vi "HoodPID.vi"(4 "Deadband":dbl, 5 "TAReset":bool, 6 "TAGains":T1={"proportional gain (Kc)"=1.0, "integral time (Ti, min)"=0.01, "derivative time (Td, min)"=0.0} {"derivative time (Td, min)" format="%.3f"; "integral time (Ti, min)" format="%.3f"; "proportional gain (Kc)" format="%.3f"}, 7 "TARange":cluster{"output high":dbl, "output low":dbl}={"output high"=0.6, "output low"=-0.6} {"output low" format="%.2f"; "output high" format="%.2f"}, 8 "TADisable Range":dbl, 9 "TAIntegral Range":dbl=10000.0, 10 "TAProcess variable":dbl, 11 "TASetpoint":dbl) -> (2 "TAoutput":dbl format="%.2f")   [LabVIEW 2020]
uses:
  <vilib>/addons/control/pid/pid.llb/PID (DBL).vi
  <vilib>/addons/control/pid/NI_PID_pid.lvlib
panel:
  out "TAChart":cluster{"Setpoint":dbl, "Process variable":dbl}(graph)
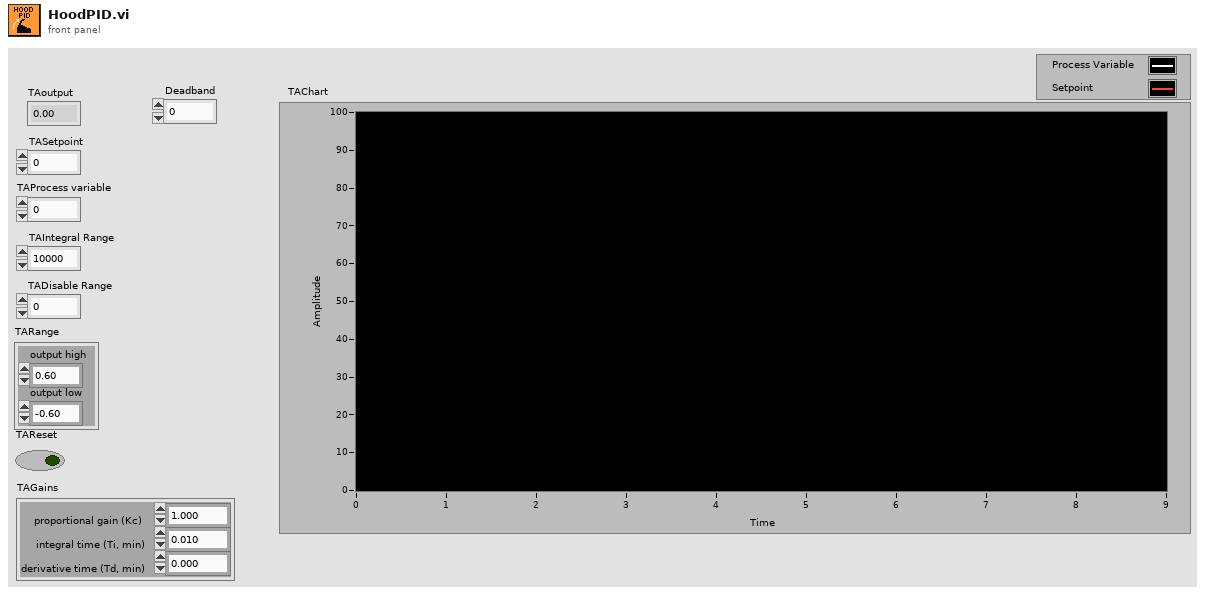
[diagram p1: front panel]
types:
  T1 = cluster{"proportional gain (Kc)":dbl, "integral time (Ti, min)":dbl, "derivative time (Td, min)":dbl}
  T2 = cluster{"TASetpoint":dbl, "TAProcess variable":dbl}
  T3 = cluster{"proportional gain (Kc)":dbl, "f":dbl, "derivative time (Td, min)":dbl}
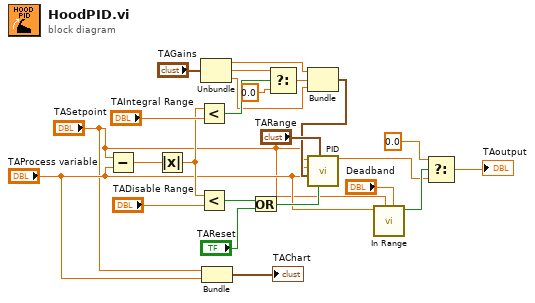
[diagram p0: block diagram]
diagram:
  n1 = Subtract(x="TASetpoint", y="TAProcess variable") -> (x-y=w23:dbl)
  n2 = Absolute Value(x=w23) -> (abs(x)=w13:dbl)
  n3 = Less?(x=w13, y="TAIntegral Range") -> (x < y?=w21:bool)
  n4 = Less?(x=w13, y="TADisable Range") -> (x < y?=w11:bool)
  n5 = Unbundle("TAGains") -> ("proportional gain (Kc)"=w16:dbl, "integral time (Ti, min)"=w19:dbl, "derivative time (Td, min)"=w15:dbl)
  n6 = Bundle("TASetpoint"="TASetpoint", "TAProcess variable"="TAProcess variable") -> (→"TAChart":T2)  [unwired: 1 in]
  n7 = Or(x=w11, y="TAReset") -> (x .or. y?=w10:bool)
  n8 = Select(t=w19, s=w21, f=0.0) -> (s? t:f=w17:dbl)
  n9 = Bundle("proportional gain (Kc)"=w16, "f"=w17, "derivative time (Td, min)"=w15) -> (w9:T3)  [unwired: 1 in]
  n10 = call-poly <vilib>:"PID.vi"("reinitialize? (F)"=w10, "output range"="TARange", "PID gains"=w9, "process variable"="TAProcess variable", "setpoint"="TASetpoint") -> ("output"=w2:dbl)  [unwired: 5 in, 1 out]
  n11 = call "In Range.vi"("Range"="Deadband", "Setpoint"="TASetpoint", "Value"="TAProcess variable") -> ("in range?"=w7:bool)  [unwired: 8 in]
  n12 = Select(t=0.0, s=w7, f=w2) -> (s? t:f=→"TAoutput":dbl)
